vi "Modbus Write.vi"(8 "Error In":errorcluster, 10 "Write Buffer":T1={"ID"="\u0001", "Function Code"="\u0003", "Length (High)"="\u0000", "Length (Low)"=",", "Start Address (High)"="\u0000", "Start Address (Middle High)"="\u0000", "Start Address (Middle Low)"="\u0010", "Start Address (Low)"="\u0000", "Data"="\u0000"}, 11 "VISA resource name":refnum<visa-resource-name>) -> (0 "Error Out":errorcluster, 3 "VISA resource name out":refnum<visa-resource-name>)   [LabVIEW 2013]
panel:
  out "read buffer":string
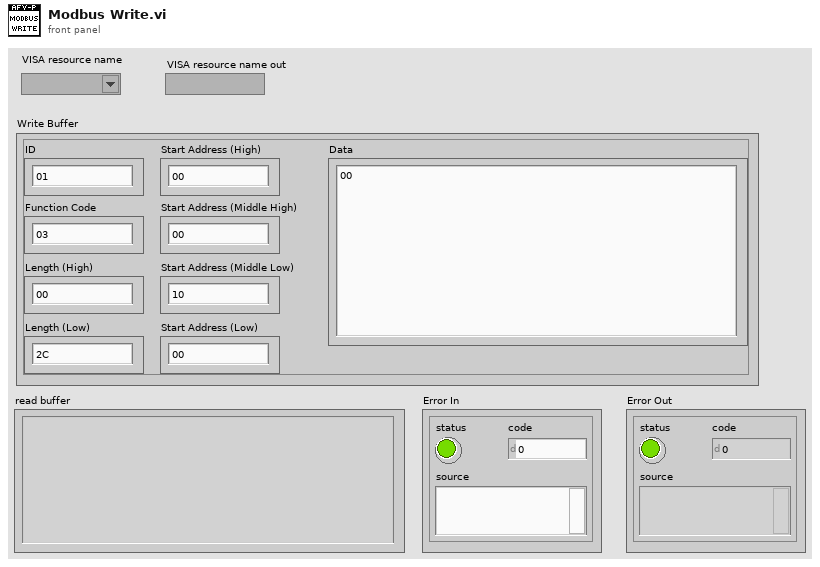
[diagram p1: front panel]
types:
  T1 = cluster{"ID":string, "Function Code":string, "Length (High)":string, "Length (Low)":string, "Start Address (High)":string, "Start Address (Middle High)":string, "Start Address (Middle Low)":string, "Start Address (Low)":string, "Data":string}
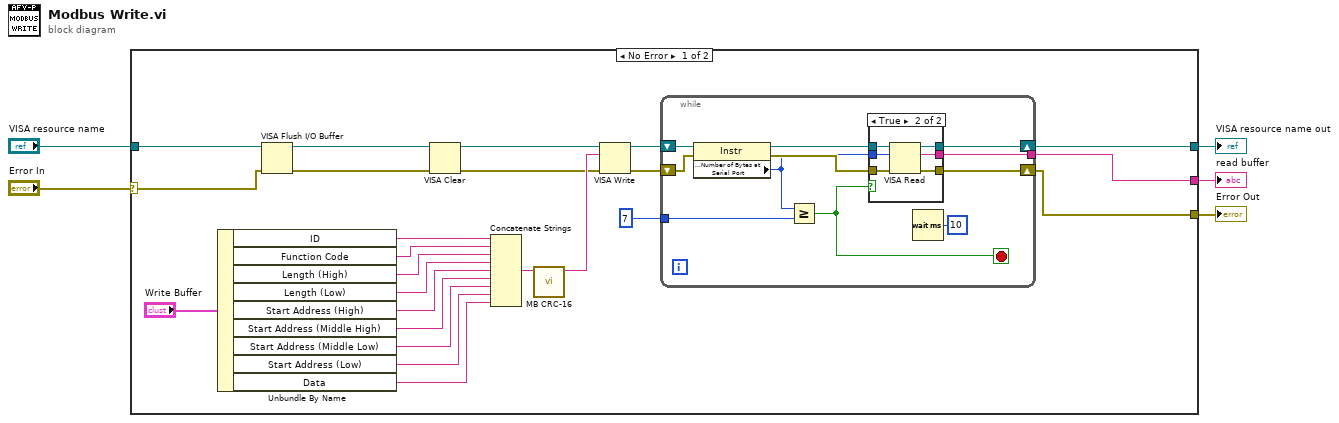
[diagram p0: block diagram]
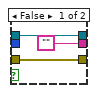
[diagram p2: hidden frame]
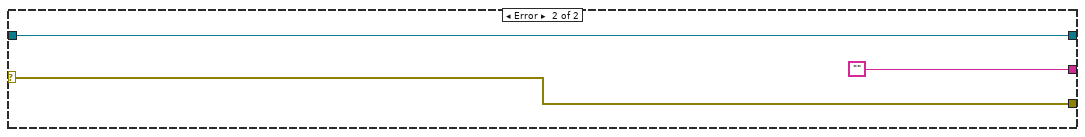
[diagram p3: hidden frame]
diagram:
  n1 = case shown="No Error" "Error In" {
    selector: "Error In" -> [w7 w52]
    tunnel: [w14 ""] -> w5
    tunnel: [w13 w52] -> w3
    tunnel: "VISA resource name" -> [w9 w50]
    tunnel: [w12 w50] -> w1
    frame No Error {
      n2 = Unbundle By Name("Write Buffer") -> ("ID"=w23:string, "Function Code"=w19:string, "Length (High)"=w24:string, "Length (Low)"=w25:string, "Start Address (High)"=w26:string, "Start Address (Middle High)"=w27:string, "Start Address (Middle Low)"=w28:string, "Start Address (Low)"=w29:string, "Data"=w20:string)
      n3 = VISA Flush I/O Buffer(VISA resource name=w9, error in (no error)=w7) -> (VISA resource name out=w10:refnum<visa-resource-name>, error out=w11:errorcluster)  [unwired: 1 in]
      n4 = VISA Clear(VISA resource name=w10, error in (no error)=w11) -> (VISA resource name out=w8:refnum<visa-resource-name>, error out=w6:errorcluster)
      n5 = Concatenate Strings(w23, w19, w24, w25, w26, w27, w28, w29, w20) -> (w21:string)
      n6 = call "MB CRC-16.vi"("String"=w21) -> ("String & CRC-16"=w18:string)  [unwired: 8 in, 2 out]
      n7 = VISA Write(VISA resource name=w8, write buffer=w18, error in (no error)=w6) -> (VISA resource name out=w16:refnum<visa-resource-name>, error out=w17:errorcluster)  [unwired: 1 out]
      n8 = while {
        tunnel: [w37] -> w14
        tunnel: u32 7 ("y") -> [w36]
        shift-right: [w33] -> w12
        shift-left: w16 -> [w35]
        shift-right: [w32] -> w13
        shift-left: w17 -> [w34]
        stop <- w31 stop-if-true
        n9 = property class="Instr"(reference=w35, error in=w34) -> (reference out=w39:refnum<visa-resource-name>, error out=w38:errorcluster, "Serial Settings:Number of Bytes at Serial Port"=w30:u32)
        n10 = Greater Or Equal?(x=w30, y=w36) -> (x >= y?=w31:bool)
        n11 = case shown="True" w31 {
          tunnel: w39 -> [w42 w49]
          tunnel: w38 -> [w41 w48]
          tunnel: w30 -> [_ w47]
          tunnel: ["" w46] -> w37
          tunnel: [w42 w45] -> w33
          tunnel: [w41 w44] -> w32
          frame False {
          }
          frame True {
            n12 = VISA Read(VISA resource name=w49, byte count=w47, error in (no error)=w48) -> (VISA resource name out=w45:refnum<visa-resource-name>, read buffer=w46:string, error out=w44:errorcluster)  [unwired: 1 out]
          }
        }
        n13 = Wait (ms)(milliseconds to wait=u32 10) -> ()  [unwired: 1 out]
      }
    }
    frame Error {
    }
  }
  "read buffer" <- w5
  "Error Out" <- w3
  "VISA resource name out" <- w1
